vi "setObjectPrivateData__ogtk.vi"(7 "error in (no error)":errorcluster, 9 "privateData":variant[](array[variant]), 10 "object in":refnum<class>) -> (0 "error out":errorcluster, 3 "object out":refnum<class>)   [LabVIEW 2023, in "openg_variant.lvlib" / "Reflection__ogtk.lvclass"]
doc: "Applies 'privateData' to the input object where privateData is an array of Variants where each element is the cluster of private data for a class in the hierarchy. \n\nGCraftsman JSON Object Serialization Toolkit\nwww.GCraftsman.com\nCopyright (c) 2017, GCraftsman"
uses:
  Reflection__ogtk.lvclass
panel:
  # "EXPERIMENTAL"
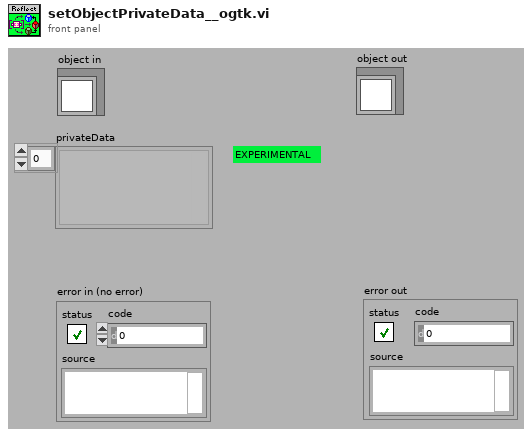
[diagram p1: front panel]
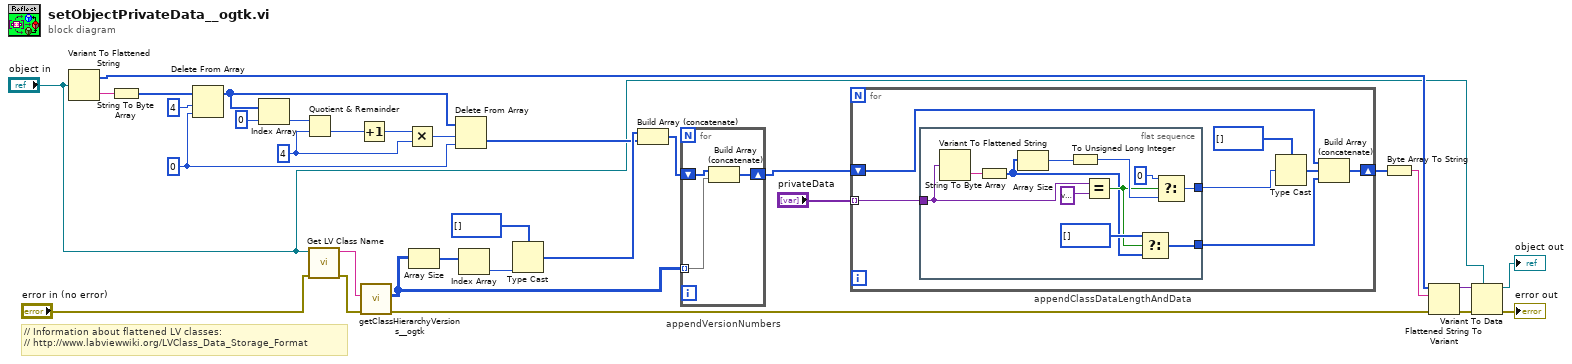
[diagram p0: block diagram]
diagram:
  w23 = u8 4 ("y")
  w30 = 0 ("index")
  # "// Information about flattened LV classes:\n// http://www.labviewwiki.org/LVClass_Data_Storage_Format"
  n1 = Variant To Flattened String(Variant="object in") -> (data string=w32:string, 1:w22:i16[])
  n2 = String To Byte Array(string=w32) -> (unsigned byte array=w29:u8[])
  n3 = Delete From Array(array=w29, length=4 ("offset (0)"), index=w30) -> (array with subset deleted=w31:u8[])  [unwired: 1 out]
  n4 = Index Array(array=w31, index=0) -> (element=w26:u8)
  n5 = Quotient & Remainder(x=w26, y=w23) -> (floor(x/y)=w25:u8)  [unwired: 1 out]
  n6 = call <vilib>:"Get LV Class Name.vi"("error in (no error)"="error in (no error)", "object"="object in") -> ("error out"=w1:errorcluster, "class name"=w7:string)  [unwired: 8 in]
  n7 = Increment(x=w25) -> (x+1=w24:u8)
  n8 = call "getClassHierarchyVersions__ogtk.vi"("error in (no error)"=w1, "className"=w7) -> ("error out"=w9:errorcluster, "allClassVersionNumbers"=w4:u8[][])  [unwired: 8 in]
  n9 = Multiply(x=w24, y=w23) -> (x*y=w21:u8)
  n10 = Array Size(array=w4) -> (size(s)=w3:i32[])
  n11 = Delete From Array(array=w31, length=w21, index=w30) -> (deleted portion=w15:u8[])  [unwired: 1 out]
  n12 = Index Array(array=w3) -> (element=w2:i32)  [unwired: 1 in]
  n13 = Type Cast(type=u8[] [] ("unsigned byte array"), x=w2) -> (*(type *) &x=w16:u8[])
  n14 = Build Array (concatenate)(w16, w15) -> (w12:u8[])
  n15 = for "appendVersionNumbers" {
    shift-right: [w33] -> w11
    shift-left: w12 -> [w34]
    tunnel: w4 -> [w35] mode=indexing
    n16 = Build Array (concatenate)(w34, w35) -> (w33:u8[])
  }
  n17 = for "appendClassDataLengthAndData" {
    shift-right: [w41] -> w14
    shift-left: w11 -> [w42]
    tunnel: "privateData" -> [w36] mode=indexing
    n18 = flat-sequence {
      tunnel: [w45] -> w38
      tunnel: [w44] -> w37
      tunnel: w36 -> [w43]
      frame #0 {
        n19 = Variant To Flattened String(Variant=w43) -> (data string=w46:string)  [unwired: 1 out]
        n20 = String To Byte Array(string=w46) -> (unsigned byte array=w48:u8[])
        n21 = Array Size(array=w48) -> (size(s)=w51:i32)
        n22 = To Unsigned Long Integer(number=w51) -> (unsigned 32bit integer=w52:u32)
        n23 = Equal?(x=w43, y=variant ("element")) -> (x = y?=w49:bool)
        n24 = Select(t=u8[] [], s=w49, f=w48) -> (s? t:f=w44:u8[])
        n25 = Select(t=u32 0, s=w49, f=w52) -> (s? t:f=w45:u32)
      }
    }
    n26 = Type Cast(type=u8[] [] ("unsigned byte array"), x=w38) -> (*(type *) &x=w39:u8[])
    n27 = Build Array (concatenate)(w42, w39, w37) -> (w41:u8[])
  }
  n28 = Byte Array To String(unsigned byte array=w14) -> (string=w13:string)
  n29 = Flattened String To Variant(4:w9, 6:w13, 7:w22) -> (0:w10:errorcluster, 3:w18:variant)
  n30 = Variant To Data(error in=w10, type="object in", Variant=w18) -> (data=→"object out":refnum<class>, error out=→"error out":errorcluster)
